vi "步响应t0t1t2.vi"(3 "步响应计算参数 in":T1, 5 "行程 in":dbl[](array[numeric])) -> (0 "步响应计算参数 out":T1, 2 "行程 out":dbl[](array[numeric]))   [LabVIEW 2013]
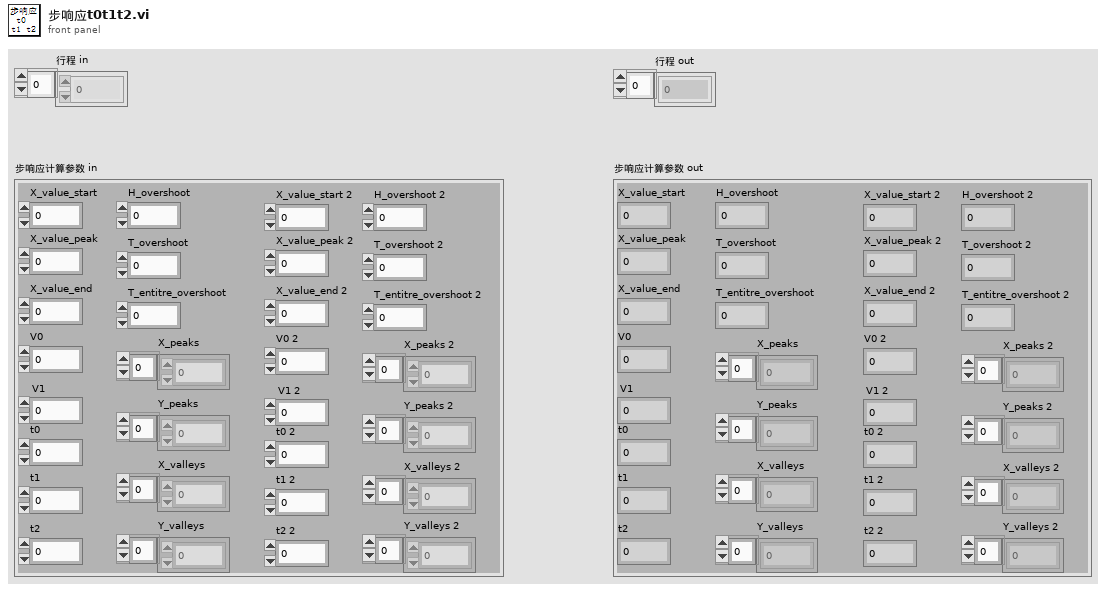
[diagram p1: front panel]
types:
  T1 = cluster{"X_value_start":dbl, "X_value_peak":dbl, "t1":dbl, "X_value_end":dbl, "V0":dbl, "V1":dbl, "t0":dbl, "X_peaks":dbl[], "X_valleys":dbl[], "Y_peaks":dbl[], "Y_valleys":dbl[], "t2":dbl, "H_overshoot":dbl, "T_overshoot":dbl, "T_entitre_overshoot":dbl, "X_value_start 2":dbl, "X_value_peak 2":dbl, "t1 2":dbl, "X_value_end 2":dbl, "V0 2":dbl, "V1 2":dbl, "t0 2":dbl, "X_peaks 2":dbl[], "X_valleys 2":dbl[], "Y_peaks 2":dbl[], "t2 2":dbl, "H_overshoot 2":dbl, "T_overshoot 2":dbl, "T_entitre_overshoot 2":dbl, "Y_valleys 2":dbl[]}
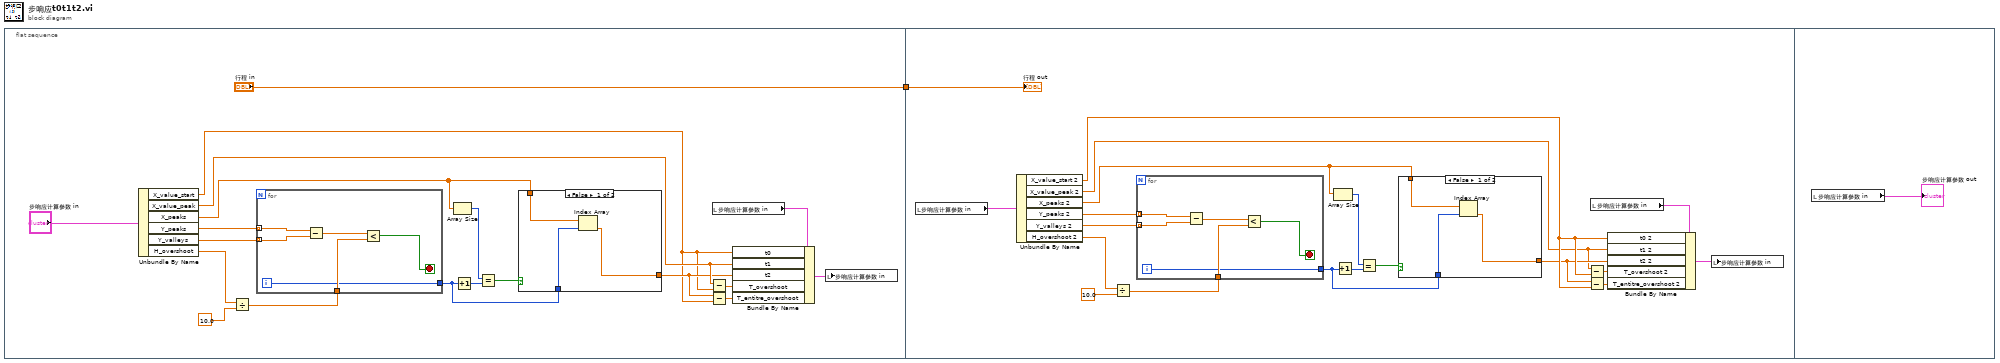
[diagram p0: block diagram]
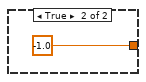
[diagram p2: hidden frame]
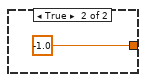
[diagram p3: hidden frame]
diagram:
  n1 = flat-sequence {
    tunnel: ["行程 in"] -> w1
    tunnel: w1 -> [w33]
    frame #0 {
      n2 = Unbundle By Name("步响应计算参数 in") -> ("X_value_start"=w5:dbl, "X_value_peak"=w8:dbl, "X_peaks"=w11:dbl[], "Y_peaks"=w13:dbl[], "Y_valleys"=w12:dbl[], "H_overshoot"=w10:dbl)
      n3 = Divide(x=w10, y=10.0) -> (x/y=w19:dbl)
      n4 = for {
        tunnel: w13 -> [w30] mode=indexing
        tunnel: w12 -> [w29] mode=indexing
        tunnel: w19 -> [w27]
        tunnel: [w25] -> w15
        i -> [w25]
        stop <- w26 stop-if-true
        n5 = Subtract(x=w30, y=w29) -> (x-y=w28:dbl)
        n6 = Less?(x=w28, y=w27) -> (x < y?=w26:bool)
      }
      n7 = Array Size(array=w11) -> (size(s)=w18:i32)
      n8 = Increment(x=w15) -> (x+1=w16:i32)
      n9 = Equal?(x=w18, y=w16) -> (x = y?=w17:bool)
      n10 = case shown="False" w17 {
        tunnel: [w21 -1.0] -> w6
        tunnel: w11 -> [w23 _]
        tunnel: w15 -> [w22 _]
        frame False {
          n11 = Index Array(array=w23, index=w22) -> (element=w21:dbl)
        }
        frame True {
        }
      }
      n12 = Subtract(x=w8, y=w5) -> (x-y=w9:dbl)
      n13 = Subtract(x=w6, y=w5) -> (x-y=w7:dbl)
      n14 = local read "步响应计算参数 in"() -> (w4:T1)
      n15 = Bundle By Name(cluster=w4, "t0"=w5, "t1"=w8, "t2"=w6, "T_overshoot"=w9, "T_entitre_overshoot"=w7) -> (w2:T1)
      n16 = local write "步响应计算参数 in"(w2) -> ()
    }
    frame #1 {
      n17 = local read "步响应计算参数 in"() -> (w32:T1)
      n18 = Unbundle By Name(w32) -> ("X_value_start 2"=w49:dbl, "X_value_peak 2"=w46:dbl, "X_peaks 2"=w43:dbl[], "Y_peaks 2"=w41:dbl[], "Y_valleys 2"=w42:dbl[], "H_overshoot 2"=w44:dbl)
      n19 = Divide(x=w44, y=10.0) -> (x/y=w36:dbl)
      n20 = for {
        tunnel: w41 -> [w59] mode=indexing
        tunnel: w42 -> [w58] mode=indexing
        tunnel: w36 -> [w56]
        tunnel: [w54] -> w40
        i -> [w54]
        stop <- w55 stop-if-true
        n21 = Subtract(x=w59, y=w58) -> (x-y=w57:dbl)
        n22 = Less?(x=w57, y=w56) -> (x < y?=w55:bool)
      }
      n23 = Array Size(array=w43) -> (size(s)=w37:i32)
      n24 = Increment(x=w40) -> (x+1=w39:i32)
      n25 = Equal?(x=w37, y=w39) -> (x = y?=w38:bool)
      n26 = case shown="False" w38 {
        tunnel: [w50 -1.0] -> w48
        tunnel: w43 -> [w52 _]
        tunnel: w40 -> [w51 _]
        frame False {
          n27 = Index Array(array=w52, index=w51) -> (element=w50:dbl)
        }
        frame True {
        }
      }
      n28 = Subtract(x=w46, y=w49) -> (x-y=w45:dbl)
      n29 = Subtract(x=w48, y=w49) -> (x-y=w47:dbl)
      n30 = local read "步响应计算参数 in"() -> (w34:T1)
      n31 = Bundle By Name(cluster=w34, "t0 2"=w49, "t1 2"=w46, "t2 2"=w48, "T_overshoot 2"=w45, "T_entitre_overshoot 2"=w47) -> (w31:T1)
      n32 = local write "步响应计算参数 in"(w31) -> ()
      "行程 out" <- w33
    }
    frame #2 {
      n33 = local read "步响应计算参数 in"() -> (→"步响应计算参数 out":T1)
    }
  }
